vi "demo.vi"() -> ()   [LabVIEW 2016]
uses:
  ZebraTable.lvlibp/XControl 1.xctl
panel:
  in  "XControl 1":string[][](xcontrol)
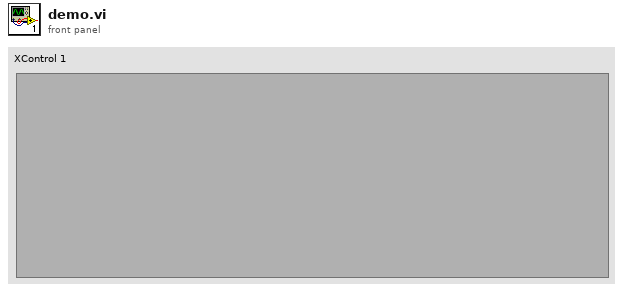
[diagram p1: front panel]
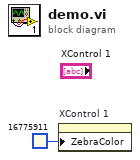
[diagram p0: block diagram]
diagram:
  n1 = property on="XControl 1" class="XControl 1 (strict)"("ZebraColor"=u32 16775911) -> ()  [unwired: 2 in, 2 out]
